vi "Bridge Balance State Machine.vi"(11 "Gyro State":i64) -> (3 "Motor Power":dbl)   [LabVIEW 2011]
uses:
  Robot Global Data.vi
  <vilib>/addons/control/pid/pid.llb/PID (DBL).vi
  <vilib>/addons/control/pid/NI_PID_pid.lvlib
panel:
  in  "PID Coerce":dbl=0.7
  in  "Bal Tol":dbl=2.0
  out "Balance":cluster{"setpoint":dbl, "GYRO":dbl}(graph)
  in  "K Derivative":dbl(knob) scale=0.0..0.01
  in  "K Integral":dbl(knob) scale=0.0..0.01
  in  "K Proportional":dbl(knob)=0.04344962855688665 scale=0.0..1.0
  in  "State -1, Bridge Tipped Down":dbl=-0.15
  in  "State 2, Fully on Bridge":dbl=0.7
  in  "State 1, Transitioning onto Bridge":dbl=0.55
  in  "State 0, Robot on Bridge":dbl
  in  "State 0, Not on Bridge":dbl=0.5
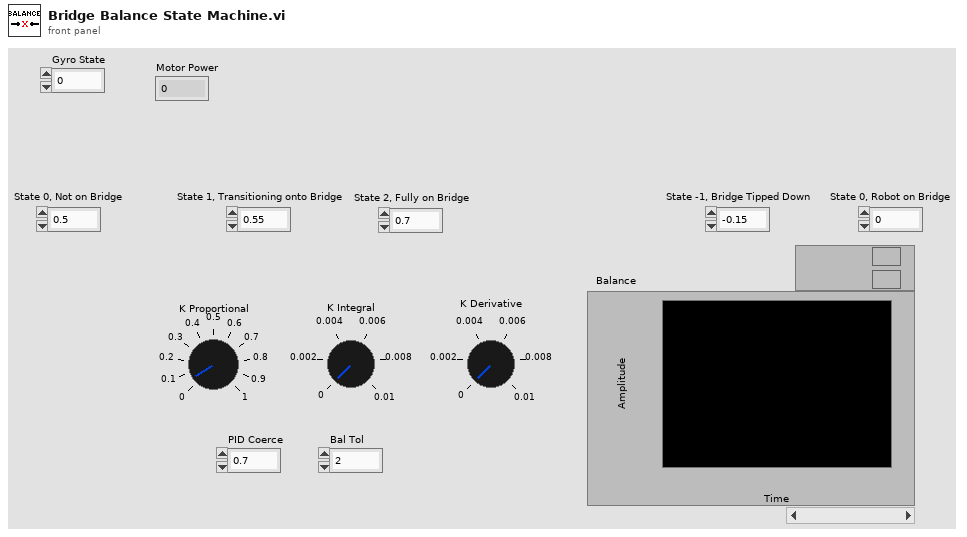
[diagram p1: front panel]
types:
  T1 = cluster{"K Proportional":dbl, "K Integral":dbl, "K Derivative":dbl}
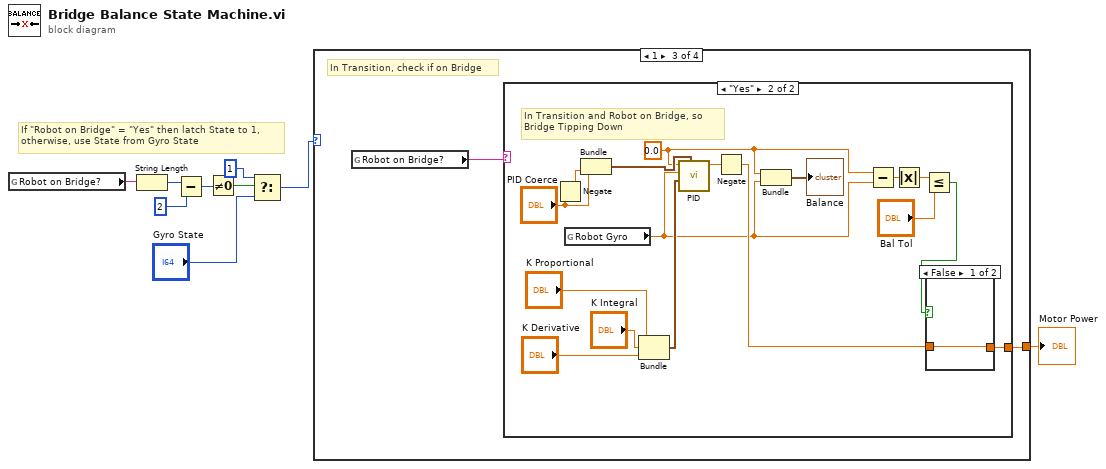
[diagram p0: block diagram]
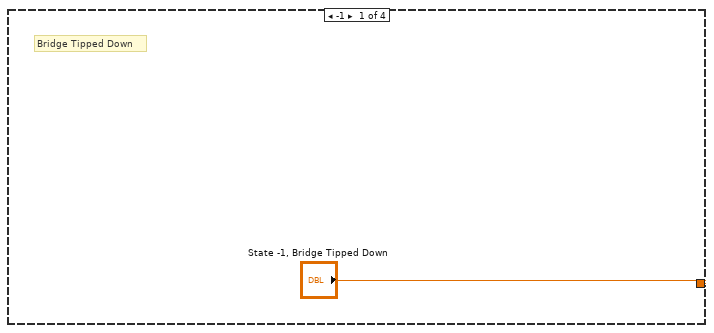
[diagram p2: hidden frame]
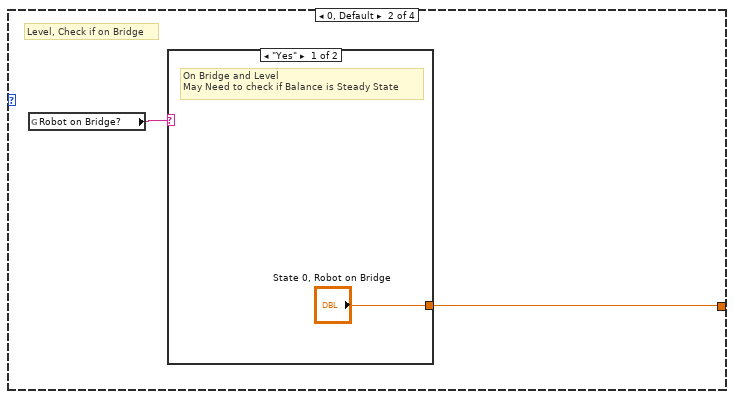
[diagram p3: hidden frame]
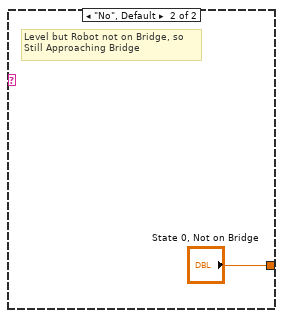
[diagram p4: hidden frame]
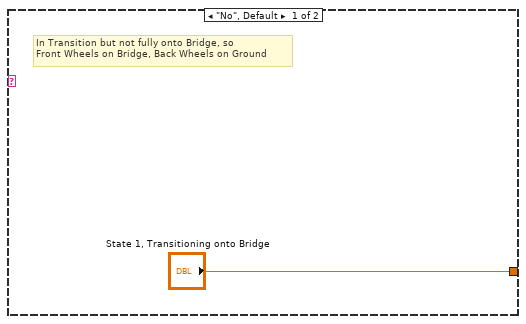
[diagram p5: hidden frame]
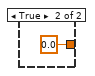
[diagram p6: hidden frame]
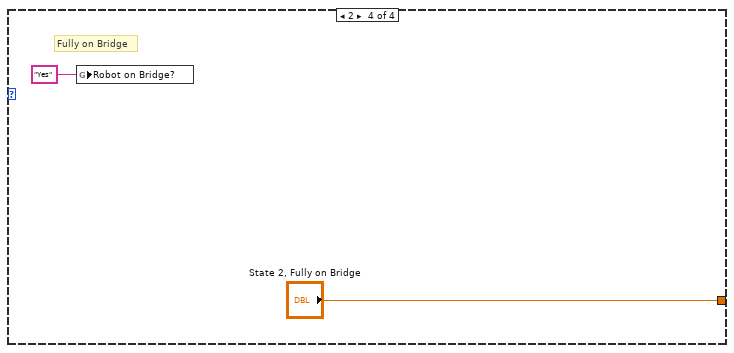
[diagram p7: hidden frame]
diagram:
  # "If \"Robot on Bridge\" = \"Yes\" then latch State to 1, \notherwise, use State from Gyro State"
  n1 = global read "Robot Global Data.vi" "Robot on Bridge?"() -> (w8:string)
  n2 = String Length(string=w8) -> (length=w7:i32)
  n3 = Subtract(x=w7, y=2) -> (x-y=w5:i32)
  n4 = Not Equal To 0?(x=w5) -> (x != 0?=w4:bool)
  n5 = Select(t=1, s=w4, f="Gyro State") -> (s? t:f=w1:i64)
  n6 = case shown="1" w1 {
    tunnel: ["State -1, Bridge Tipped Down" w12 w16 "State 2, Fully on Bridge"] -> w9
    frame -1 {
      # "Bridge Tipped Down"
    }
    frame 0, Default {
      # "Level, Check if on Bridge"
      n7 = global read "Robot Global Data.vi" "Robot on Bridge?"() -> (w11:string)
      n8 = case shown="\"Yes\"" w11 {
        tunnel: ["State 0, Robot on Bridge" "State 0, Not on Bridge"] -> w12
        frame "Yes" {
          # "On Bridge and Level\nMay Need to check if Balance is Steady State"
        }
        frame "No", Default {
          # "Level but Robot not on Bridge, so\nStill Approaching Bridge"
        }
      }
    }
    frame 1 {
      # "In Transition, check if on Bridge"
      n9 = global read "Robot Global Data.vi" "Robot on Bridge?"() -> (w15:string)
      n10 = case shown="\"Yes\"" w15 {
        tunnel: ["State 1, Transitioning onto Bridge" w18] -> w16
        frame "No", Default {
          # "In Transition but not fully onto Bridge, so\nFront Wheels on Bridge, Back Wheels on Ground"
        }
        frame "Yes" {
          w22 = 0.0 ("setpoint")
          # "In Transition and Robot on Bridge, so \nBridge Tipping Down"
          n11 = Negate(x="PID Coerce") -> (-x=w32:dbl)
          n12 = global read "Robot Global Data.vi" "Robot Gyro"() -> (w21:dbl)
          n13 = Bundle("PID Coerce"="PID Coerce", w32) -> (w34:cluster{"PID Coerce":dbl, dbl})  [unwired: 1 out]
          n14 = Bundle("K Proportional"="K Proportional", "K Integral"="K Integral", "K Derivative"="K Derivative") -> (w30:T1)  [unwired: 1 out]
          n15 = call-poly <vilib>:"PID.vi"("output range"=w34, "PID gains"=w30, "process variable"=w21, "setpoint"=w22) -> ("output"=w31:dbl)  [unwired: 6 in, 1 out]
          n16 = Negate(x=w31) -> (-x=w26:dbl)
          n17 = Bundle("setpoint"=w22, "Robot Gyro"=w21) -> (→"Balance":cluster{"setpoint":dbl, "Robot Gyro":dbl})  [unwired: 1 out]
          n18 = Subtract(x=w22, y=w21) -> (x-y=w24:dbl)
          n19 = Absolute Value(x=w24) -> (abs(x)=w23:dbl)
          n20 = Less Or Equal?(x=w23, y="Bal Tol") -> (x <= y?=w19:bool)
          n21 = case shown="False" w19 {
            tunnel: w26 -> [w35 _]
            tunnel: [w35 0.0 ("State 1, Bridge Tipping Down")] -> w18
            frame False {
            }
            frame True {
            }
          }
        }
      }
    }
    frame 2 {
      # "Fully on Bridge"
      n22 = global write "Robot Global Data.vi" "Robot on Bridge?"("Yes" ("Robot on Bridge?")) -> ()
    }
  }
  "Motor Power" <- w9
